vi "Run.vi"(8 "error in (no error)":errorcluster, 10 "Enum":enum16{"Bacward", "Forward", "Release"}(ring), 11 "DCMotor in":refnum<class "DCMotor.lvclass">) -> (0 "error out":errorcluster, 3 "DCMotor out":refnum<class "DCMotor.lvclass">)   [LabVIEW 2022 SP3, in "Motorshield.lvlib" / "DCMotor.lvclass"]
uses:
  DCMotor.lvclass
  C:/Users/Carlos/Desktop/onlab/source/Motorshield/Motorshield/Motorshield.lvclass
  DCMotor.lvclass/DCMotor.ctl
  Motorshield/Motorshield.lvclass
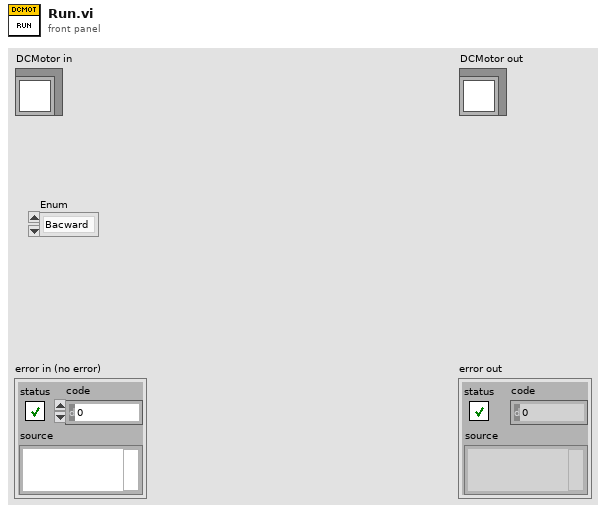
[diagram p1: front panel]
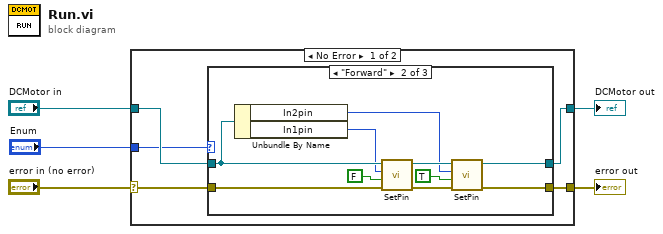
[diagram p0: block diagram]
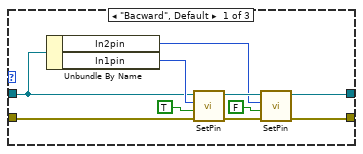
[diagram p2: hidden frame]
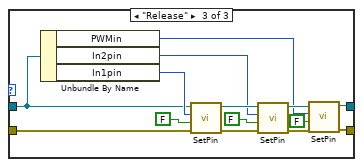
[diagram p3: hidden frame]
diagram:
  n1 = case shown="No Error" "error in (no error)" {
    selector: "error in (no error)" -> [w10 w46]
    tunnel: [w9 w46] -> w4
    tunnel: [w8 w45] -> w2
    tunnel: "DCMotor in" -> [w7 w45]
    tunnel: "Enum" -> [w6 _]
    frame No Error {
      n2 = case shown="\"Forward\"" w6 {
        tunnel: w10 -> [w13 w30 w38]
        tunnel: [w12 w28 w33] -> w9
        tunnel: [w11 w27 w34] -> w8
        tunnel: w7 -> [w14 w25 w37]
        frame "Bacward", Default {
          n3 = Unbundle By Name(w14) -> ("In2pin"=w17:u8, "In1pin"=w18:u8)
          n4 = call "SetPin.vi"("error in (no error)"=w13, "Value"=TRUE, "Led num"=w18, "Motorshield in"=w14) -> ("error out"=w20:errorcluster, "Motorshield out"=w19:refnum<class "DCMotor.lvclass">)  [unwired: 6 in]
          n5 = call "SetPin.vi"("error in (no error)"=w20, "Value"=FALSE, "Led num"=w17, "Motorshield in"=w19) -> ("error out"=w12:errorcluster, "Motorshield out"=w11:refnum<class "DCMotor.lvclass">)  [unwired: 6 in]
        }
        frame "Forward" {
          n6 = Unbundle By Name(w25) -> ("In2pin"=w23:u8, "In1pin"=w24:u8)
          n7 = call "SetPin.vi"("error in (no error)"=w30, "Value"=FALSE, "Led num"=w24, "Motorshield in"=w25) -> ("error out"=w29:errorcluster, "Motorshield out"=w26:refnum<class "DCMotor.lvclass">)  [unwired: 6 in]
          n8 = call "SetPin.vi"("error in (no error)"=w29, "Value"=TRUE, "Led num"=w23, "Motorshield in"=w26) -> ("error out"=w28:errorcluster, "Motorshield out"=w27:refnum<class "DCMotor.lvclass">)  [unwired: 6 in]
        }
        frame "Release" {
          n9 = Unbundle By Name(w37) -> ("PWMin"=w32:u8, "In2pin"=w41:u8, "In1pin"=w42:u8)
          n10 = call "SetPin.vi"("error in (no error)"=w38, "Value"=FALSE, "Led num"=w42, "Motorshield in"=w37) -> ("error out"=w44:errorcluster, "Motorshield out"=w43:refnum<class "DCMotor.lvclass">)  [unwired: 6 in]
          n11 = call "SetPin.vi"("error in (no error)"=w44, "Value"=FALSE, "Led num"=w41, "Motorshield in"=w43) -> ("error out"=w36:errorcluster, "Motorshield out"=w35:refnum<class "DCMotor.lvclass">)  [unwired: 6 in]
          n12 = call "SetPin.vi"("error in (no error)"=w36, "Value"=FALSE, "Led num"=w32, "Motorshield in"=w35) -> ("error out"=w33:errorcluster, "Motorshield out"=w34:refnum<class "DCMotor.lvclass">)  [unwired: 6 in]
        }
      }
    }
    frame Error {
    }
  }
  "error out" <- w4
  "DCMotor out" <- w2
